vi "Launch Async Auth.vi"(5 "Refresh Only?":bool, 6 "Failed HTML Response":refnum<class "Response.lvclass">, 7 "Success Response":refnum<class "Response.lvclass">, 8 "error in (no error)":errorcluster, 9 "Timeout S (60)":dbl=60.0, 10 "Authorization in":refnum<class "Authorization.lvclass">, 11 "OAuth2 in":refnum<class "OAuth2.lvclass">) -> (0 "error out":errorcluster, 1 "Async Authentication":refnum<class "Async Authorization.lvclass">, 3 "OAuth2 out":refnum<class "OAuth2.lvclass">)   [LabVIEW 2020, in "OAuth2.lvlib" / "OAuth2.lvclass"]
uses:
  OAuth2.lvclass
  Auth Async.vi
  Async Authorization/Async Authorization.lvclass
  Authorization/Authorization.lvclass
  <vilib>/IlluminatedG/IG HTTP Utils/HTTP Utils/Response/Response.lvclass
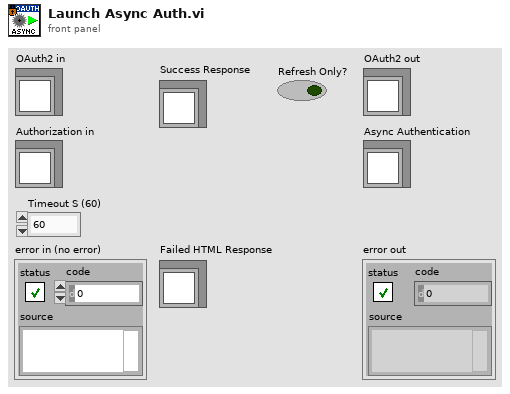
[diagram p1: front panel]
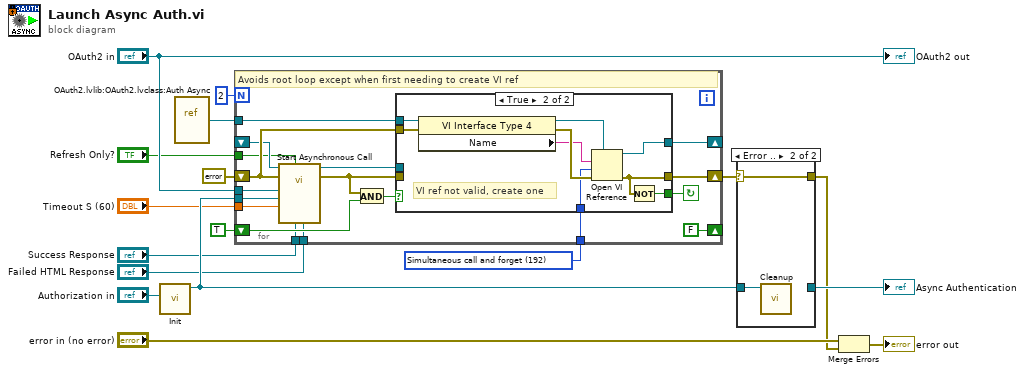
[diagram p0: block diagram]
diagram:
  w14 = 192 items=["Record modifications"=1, "Open templates for editing"=2, "Prompt user to save"=4, "Prepare for reentrant run"=8, "Prompt to find missing subVIs"=16, "Hide loading dialog box"=32, "Enable simultaneous calls"=64, "Prepare to call and forget"=128, "Simultaneous call and forget"=192, "Prepare to call and collect"=256, "Simultaneous call and collect"=320]
  n1 = call "Init.vi"("Authorization"="Authorization in") -> ("Async Authorization out"=w8:refnum<class "Async Authorization.lvclass">)  [unwired: 9 in, 1 out]
  n2 = vi-ref "OAuth2.lvlib:OAuth2.lvclass:Auth Async.vi"() -> (w13:refnum<vi>)
  n3 = for {
    N: 2 -> [_]
    tunnel: w13 -> [w34]
    tunnel: w14 -> [w33]
    shift-right: [w32] -> _
    shift-left: _ -> [w31]
    shift-right: [w29] -> w9
    shift-left: errorcluster {"status"=FALSE, "code"=0, "source"=""} ("error constant") -> [w35]
    shift-right: [FALSE] -> _
    shift-left: TRUE -> [w26]
    tunnel: "OAuth2 in" -> [w23]
    tunnel: w8 -> [w22]
    tunnel: "Timeout S (60)" -> [w21]
    tunnel: "Refresh Only?" -> [w20]
    tunnel: "Success Response" -> [w19]
    tunnel: "Failed HTML Response" -> [w18]
    stop <- w25 continue-if-true
    # "Avoids root loop except when first needing to create VI ref"
    n4 = call-by-ref "Start Asynchronous Call"(reference=w31, error in=w35, "Failed Response"=w18, "Complete Response"=w19, "Refresh Only?"=w20, "Timeout S"=w21, "Async Authorization"=w22, "OAuth2 in"=w23) -> (reference out=w30:refnum<vi>, error out=w28:errorcluster)  [unwired: 6 in]
    n5 = And(x=w28, y=w26) -> (x .and. y?=w27:bool)
    n6 = case shown="True" w27 {
      tunnel: w34 -> [_ w45]
      tunnel: w33 -> [_ w43]
      tunnel: [w37 w41] -> w32
      tunnel: w30 -> [w37 _]
      tunnel: [w36 w39] -> w29
      tunnel: w28 -> [w36 _]
      tunnel: w35 -> [_ w40]
      tunnel: [_ w38] -> w25
      frame False {
        # "Keep reusing valid VI ref"
      }
      frame True {
        # "VI ref not valid, create one"
        n7 = property class="VI Interface Type 4"(reference=w45, error in=w40) -> (reference out=w42:refnum<vi>, error out=w46:errorcluster, "Name"=w44:string)
        n8 = Open VI Reference(type specifier VI Refnum (for type only)=w42, vi path=w44, options=w43, error in (no error)=w46) -> (vi reference=w41:refnum<vi>, error out=w39:errorcluster)  [unwired: 2 in]
        n9 = Not(x=w39) -> (.not. x?=w38:bool)
      }
    }
  }
  n10 = case shown="Error .." w9 {
    selector: w9 -> [_ w48]
    tunnel: w8 -> [w47 w49]
    tunnel: [w47 _] -> w7
    tunnel: [_ w48] -> w5
    frame No Error {
    }
    frame Error {
      n11 = call "Cleanup.vi"("Async Authorization in"=w49) -> ()  [unwired: 10 in, 1 out]
    }
  }
  "Async Authentication" <- w7
  n12 = Merge Errors("error in (no error)", w5) -> (→"error out":errorcluster)
  "OAuth2 out" <- "OAuth2 in"
